vi "FPGA Target 2.vi"() -> ()   [LabVIEW 2025]
uses:
  <vilib>/Platform/TimedLoop/XDataNode/wakeup.ctl
  <vilib>/Platform/TimedLoop/XDataNode/XDNodeRunTimeDep.lvlib
  <vilib>/Platform/TimedLoop/XDataNode/nitl_modes.ctl
  <vilib>/Platform/TimedLoop/XDataNode/timing_clust.ctl
  <vilib>/Platform/TimedLoop/XDataNode/XDataNode.xnode
  SubModules/Engine Simulation Toolkit FPGA IP/IP Source/APU/APU.lvlib
  <vilib>/rvi/DataTransferAndStorage/Container/XNode/niFpgaContainer.xnode
  Templates/FPGA Wizard Templates.lvlib
  <vilib>/rvi/interface/RandomDataEmulation/nirviRandomDataFpgaReadWriteTemplate.vi
  SubModules/Engine Simulation Toolkit FPGA IP/IP Source/Digital Pattern Generation/Digital Pattern Generation.lvlib
  SubModules/Engine Simulation Toolkit FPGA IP/IP Source/Directional Speed/Directional Speed.lvlib
  SubModules/Engine Simulation Toolkit FPGA IP/IP Source/Analog Replay/Analog Replay.lvlib
  SubModules/FPGA Addon Speciality IO/Source/Speciality FPGA IO.lvlib
  SubModules/Engine Simulation Toolkit FPGA IP/IP Source/Knock Sensor/Knock Sensor.lvlib
  SubModules/Engine Simulation Toolkit FPGA IP/IP Source/ECU Event/Timing/ECU Event Timing.lvlib
  SubModules/Engine Simulation Toolkit FPGA IP/IP Source/ECU Event/Timing/Measure Events (Non-40MHz).vi
  SubModules/Engine Simulation Toolkit FPGA IP/IP Source/ECU Event/Timing/Capture Settings.ctl
  SubModules/Engine Simulation Toolkit FPGA IP/IP Source/APU/Shared Settings.ctl
  SubModules/Engine Simulation Toolkit FPGA IP/IP Source/Version Token.ctl
  SubModules/Engine Simulation Toolkit FPGA IP/IP Source/Engine Simulation Toolkit.lvlib
  SubModules/Engine Simulation Toolkit FPGA IP/IP Source/APU/Settings.ctl
  SubModules/Engine Simulation Toolkit FPGA IP/IP Source/APU/Input.ctl
  SubModules/Engine Simulation Toolkit FPGA IP/IP Source/APU/Output.ctl
  SubModules/Engine Simulation Toolkit FPGA IP/IP Source/Digital Pattern Generation/Load Input.ctl
  SubModules/Engine Simulation Toolkit FPGA IP/IP Source/Directional Speed/Load Input.ctl
  SubModules/Engine Simulation Toolkit FPGA IP/IP Source/Analog Replay/Load Input.ctl
  SubModules/FPGA Addon Speciality IO/Source/Types/PWM.Measure.Analog.Settings.ctl
  SubModules/FPGA Addon Speciality IO/Source/Types/PWM.Measure.Analog.Measurement.ctl
  SubModules/Engine Simulation Toolkit FPGA IP/IP Source/Knock Sensor/Cylinder Settings.ctl
  SubModules/Engine Simulation Toolkit FPGA IP/IP Source/Knock Sensor/Cylinder Input.ctl
  SubModules/Engine Simulation Toolkit FPGA IP/IP Source/Knock Sensor/Generate Settings.ctl
  SubModules/Engine Simulation Toolkit FPGA IP/IP Source/Knock Sensor/Generate Input.ctl
  SubModules/Engine Simulation Toolkit FPGA IP/IP Source/Analog Replay/Settings.ctl
  SubModules/Engine Simulation Toolkit FPGA IP/IP Source/Analog Replay/Input.ctl
  SubModules/FPGA Addon Speciality IO/Source/Types/Sine.Generate.Settings.ctl
  SubModules/FPGA Addon Speciality IO/Source/Types/PWM.Generate.Digital.Settings.ctl
  SubModules/Engine Simulation Toolkit FPGA IP/IP Source/Digital Pattern Generation/Settings.ctl
  SubModules/Engine Simulation Toolkit FPGA IP/IP Source/Digital Pattern Generation/Input.ctl
  SubModules/Engine Simulation Toolkit FPGA IP/IP Source/Directional Speed/Settings.ctl
  SubModules/Engine Simulation Toolkit FPGA IP/IP Source/Directional Speed/Input.ctl
  SubModules/FPGA Addon Speciality IO/Source/Types/WSS.Generate.Digital.Settings.ctl
  SubModules/FPGA Addon Speciality IO/Source/Types/PWM.Measure.Digital.Settings.ctl
  SubModules/FPGA Addon Speciality IO/Source/Types/PWM.Measure.Digital.Measurement.ctl
  SubModules/Engine Simulation Toolkit FPGA IP/IP Source/ECU Event/Timing/Measure Settings.ctl
  SubModules/Engine Simulation Toolkit FPGA IP/IP Source/ECU Event/Timing/Measure Output.ctl
  SubModules/Engine Simulation Toolkit FPGA IP/IP Source/ECU Event/Timing/Capture Output.ctl
  SubModules/FPGA Addon Speciality IO/Source/Types/QuadratureEncoder.Measure.Digital.Settings.ctl
  SubModules/FPGA Addon Speciality IO/Source/Types/QuadratureEncoder.Measure.Digital.Measurement.ctl
panel:
  out "Check The Channel 2":bool
  out "Check The Channel 1":bool
  out "Measured CAM Position.Measure":T1
  in  "Measured CAM Position.Settings":T2={"DIRECTION"=0, "RESET VALUE"=0, "A RESET STATE"=TRUE, "B RESET STATE"=TRUE, "Z RESET STATE"=TRUE}
  out "Measured Engine Position.Measure":T1
  in  "Measured Engine Position.Settings":T2={"DIRECTION"=0, "RESET VALUE"=0, "A RESET STATE"=TRUE, "B RESET STATE"=TRUE, "Z RESET STATE"=TRUE}
  out "Connector1 DIO Bank0.Monitor":bool[](array[boolean])
  out "capture.Cyl Inj 3.Event 4":T3
  out "capture.Cyl Inj 3.Event 3":T3
  out "capture.Cyl Inj 3.Event 2":T3
  out "capture.Cyl Inj 3.Event 1":T3
  out "status.Cyl Inj 3":T4
  in  "settings.Cyl Inj 3":T5
  out "capture.Cyl Inj 2.Event 4":T3
  out "capture.Cyl Inj 2.Event 3":T3
  out "capture.Cyl Inj 2.Event 2":T3
  out "capture.Cyl Inj 2.Event 1":T3
  out "status.Cyl Inj 2":T4
  in  "settings.Cyl Inj 2":T5
  out "capture.Cyl Inj 1.Event 4":T3
  out "capture.Cyl Inj 1.Event 3":T3
  out "capture.Cyl Inj 1.Event 2":T3
  out "capture.Cyl Inj 1.Event 1":T3
  out "status.Cyl Inj 1":T4
  in  "settings.Cyl Inj 1":T5
  out "PWM IN 2.Measure":T6
  in  "PWM IN 2.Settings":T7={"ACTIVE EDGE"=TRUE, "TIMEOUT"=40000000}
  out "PWM IN 1.Measure":T6
  in  "PWM IN 1.Settings":T7={"ACTIVE EDGE"=TRUE, "TIMEOUT"=40000000}
  out "Key State":bool
  out "Switch State":bool
  out "Relay State":bool
  out "Connector0 DIO Bank2.Monitor":bool[](array[boolean])
  out "Connector0 DIO Bank1.Monitor":bool[](array[boolean])
  in  "Read Passenger WS.Settings":T8={"ACTIVE EDGE"=TRUE, "ACTIVE TICKS"=0, "INACTIVE TICKS"=0, "DATA"=0, "SENSOR TYPE"=0}
  in  "Rear Driver WS.Settings":T8={"ACTIVE EDGE"=TRUE, "ACTIVE TICKS"=0, "INACTIVE TICKS"=0, "DATA"=0, "SENSOR TYPE"=0}
  in  "Front Passenger WS.Settings":T8={"ACTIVE EDGE"=TRUE, "ACTIVE TICKS"=0, "INACTIVE TICKS"=0, "DATA"=0, "SENSOR TYPE"=0}
  in  "Front Driver WS.Settings":T8={"ACTIVE EDGE"=TRUE, "ACTIVE TICKS"=0, "INACTIVE TICKS"=0, "DATA"=0, "SENSOR TYPE"=0}
  out "Connector0 DIO Bank0.Monitor":bool[](array[boolean])
  in  "input.Crank":T9
  in  "settings.Crank":T10
  in  "input.Crank_Temp":T11
  in  "settings.Crank_Temp":T12
  in  "Switch":bool
  in  "Key":bool
  in  "input.Exhaust CAM 1":T11
  in  "settings.Exhaust CAM 1":T12
  in  "input.Intake CAM 1":T11
  in  "settings.Intake CAM 1":T12
  in  "PWM Out 2.Settings":T13={"ACTIVE EDGE"=TRUE, "ACTIVE TICKS"=0, "INACTIVE TICKS"=0}
  in  "PWM Out 1.Settings":T13={"ACTIVE EDGE"=TRUE, "ACTIVE TICKS"=0, "INACTIVE TICKS"=0}
  out "Connector1 AO Bank0.Monitor":fxp<+/-,32,8>[](array[numeric])
  in  "Simple Knock 2.Settings":T14={"AMP"=0.0, "OFFSET"=0.0, "PERIODS/TICKS"=2.4999957531690598e-05}
  in  "Simple Knock 1.Settings":T14={"AMP"=0.0, "OFFSET"=0.0, "PERIODS/TICKS"=2.4999957531690598e-05}
  in  "input.VR Sensor2":T15
  in  "settings.VR Sensor2":T16
  in  "input.VR Sensor1":T15
  in  "settings.VR Sensor1":T16
  in  "Power Supply Setpoint":fxp<+/-,32,8> format="%#_27g"
  in  "Dyno Setpoint":fxp<+/-,32,8> format="%#_27g"
  in  "input.Knock2":T17
  in  "settings.Knock2":T18
  in  "input.Knock2.Cylinder 6":T19={"probability compare"=65535, "high freq scaler"=0.0, "trigger position"=0}
  in  "settings.Knock2.Cylinder 6":T20
  in  "input.Knock2.Cylinder 5":T19={"probability compare"=65535, "high freq scaler"=0.0, "trigger position"=0}
  in  "settings.Knock2.Cylinder 5":T20
  in  "input.Knock2.Cylinder 4":T19={"probability compare"=65535, "high freq scaler"=0.0, "trigger position"=0}
  in  "settings.Knock2.Cylinder 4":T20
  in  "input.Knock2.Cylinder 3":T19={"probability compare"=65535, "high freq scaler"=0.0, "trigger position"=0}
  in  "settings.Knock2.Cylinder 3":T20
  in  "input.Knock2.Cylinder 2":T19={"probability compare"=65535, "high freq scaler"=0.0, "trigger position"=0}
  in  "settings.Knock2.Cylinder 2":T20
  in  "input.Knock2.Cylinder 1":T19={"probability compare"=65535, "high freq scaler"=0.0, "trigger position"=0}
  in  "settings.Knock2.Cylinder 1":T20
  in  "input.Knock1":T17
  in  "settings.Knock1":T18
  in  "input.Knock1.Cylinder 6":T19={"probability compare"=65535, "high freq scaler"=0.0, "trigger position"=0}
  in  "settings.Knock1.Cylinder 6":T20
  in  "input.Knock1.Cylinder 5":T19={"probability compare"=65535, "high freq scaler"=0.0, "trigger position"=0}
  in  "settings.Knock1.Cylinder 5":T20
  in  "input.Knock1.Cylinder 4":T19={"probability compare"=65535, "high freq scaler"=0.0, "trigger position"=0}
  in  "settings.Knock1.Cylinder 4":T20
  in  "input.Knock1.Cylinder 3":T19={"probability compare"=65535, "high freq scaler"=0.0, "trigger position"=0}
  in  "settings.Knock1.Cylinder 3":T20
  in  "input.Knock1.Cylinder 2":T19={"probability compare"=65535, "high freq scaler"=0.0, "trigger position"=0}
  in  "settings.Knock1.Cylinder 2":T20
  in  "input.Knock1.Cylinder 1":T19={"probability compare"=65535, "high freq scaler"=0.0, "trigger position"=0}
  in  "settings.Knock1.Cylinder 1":T20
  out "Temp2":fxp<+/-,32,8> format="%#_27g"
  out "Temp1":fxp<+/-,32,8> format="%#_27g"
  out "Pressure4":fxp<+/-,32,8> format="%#_27g"
  out "Pressure3":fxp<+/-,32,8> format="%#_27g"
  out "Injector4.Measure":T21
  in  "Injector4.Settings":T22={"ACTIVE EDGE"=TRUE, "TIMEOUT"=40000000, "THRESHOLD"=50.0}
  out "Injector3.Measure":T21
  in  "Injector3.Settings":T22={"ACTIVE EDGE"=TRUE, "TIMEOUT"=40000000, "THRESHOLD"=50.0}
  out "Pressure2":fxp<+/-,32,8> format="%#_27g"
  out "Pressure1":fxp<+/-,32,8> format="%#_27g"
  out "Connector1 AI Bank0.Monitor":fxp<+/-,27,5>[](array[numeric])
  in  "load input.VR Sensor2":T23={"Data"=[0, 0, 0, 0, 0, 0, 0, 0, 0, 0, 0, 0, 0, 0, 0, 0], "LoadOffset"=0, "Done"=FALSE}
  in  "load input.VR Sensor1":T23={"Data"=[0, 0, 0, 0, 0, 0, 0, 0, 0, 0, 0, 0, 0, 0, 0, 0], "LoadOffset"=0, "Done"=FALSE}
  in  "load input.Crank":T24
  in  "load input.Crank_Temp":T25
  in  "load input.Exhaust CAM 1":T25
  in  "load input.Intake CAM 1":T25
  out "Actual Analog Input Loop Period (usec)":u32
  out "Actual Analog Output Loop Period (usec)":u32
  out "Actual Digital Loop Period (usec)":u32
  out "Actual DMA Loop Period (usec)":u32
  in  "Analog Input Loop Timer (uSec)":u32=10
  out "output.apu 1":T26 caption="output"
  in  "input.apu 1":T27={"desired speed"=0.0, "reset"=TRUE} caption="input"
  in  "settings.apu 1":T28 caption="settings"
  in  "est.version":T29
  in  "shared settings.apu 1":T30 {"start" format="%#.15g"}
  in  "go.apu 1":bool
  in  "Digital Loop Timer (uSec)":u32=10
  in  "Analog Output Loop Timer (uSec)":u32=10
  in  "DMA.Enable":bool
  in  "DMA.MinimumSamples":u32=100000 caption="DMA Loop Timer (uSec)"
  out "DMA.Timeout":bool
  in  "DMA.Timeout.Reset":bool
  in  "DMA Loop Timer (uSec)":u32=10
types:
  T1 = typedef "Speciality FPGA IO.lvlib/QuadratureEncoder.Measure.Digital.Measurement.ctl" = cluster{"POSITION":i32}
  T2 = typedef "Speciality FPGA IO.lvlib/QuadratureEncoder.Measure.Digital.Settings.ctl" = cluster{"DIRECTION":u8, "RESET VALUE":i32, "A RESET STATE":bool, "B RESET STATE":bool, "Z RESET STATE":bool}
  T3 = typedef "Engine Simulation Toolkit.lvlib/ECU Event Timing.lvlib/Capture Output.ctl" = cluster{"Start":u16, "End":u16, "Duration (tics)":fxp<+,18,18>, "Event present":bool}
  T4 = typedef "Engine Simulation Toolkit.lvlib/ECU Event Timing.lvlib/Measure Output.ctl" = cluster{"stuck active":bool, "window all active":bool, "window orphan start":bool, "window orphan end":bool}
  T5 = typedef "Engine Simulation Toolkit.lvlib/ECU Event Timing.lvlib/Measure Settings.ctl" = cluster{"max":u16, "min":u16, "active high":bool, "wrap":bool}
  T6 = typedef "Speciality FPGA IO.lvlib/PWM.Measure.Digital.Measurement.ctl" = cluster{"ACTIVE TICKS":u32, "INACTIVE TICKS":u32, "ACQ TICKS":u32}
  T7 = typedef "Speciality FPGA IO.lvlib/PWM.Measure.Digital.Settings.ctl" = cluster{"ACTIVE EDGE":bool, "TIMEOUT":u32}
  T8 = typedef "Speciality FPGA IO.lvlib/WSS.Generate.Digital.Settings.ctl" = cluster{"ACTIVE EDGE":bool, "ACTIVE TICKS":u32, "INACTIVE TICKS":u32, "DATA":u8, "SENSOR TYPE":u8}
  T9 = typedef "Engine Simulation Toolkit.lvlib/Directional Speed.lvlib/Input.ctl" = cluster{"td (tics)":u16, "tf (tics)":u16, "tr (tics)":u16}
  T10 = typedef "Engine Simulation Toolkit.lvlib/Directional Speed.lvlib/Settings.ctl" = cluster{"Upper Value":u16, "Lower Value":u16, "Upper Index":fxp<+,10,10>, "Lower Index":fxp<+,10,10>, "Enabled":bool}
  T11 = typedef "Engine Simulation Toolkit.lvlib/Digital Pattern Generation.lvlib/Input.ctl" = cluster{"Offset":i16}
  T12 = typedef "Engine Simulation Toolkit.lvlib/Digital Pattern Generation.lvlib/Settings.ctl" = cluster{"edge 1":u16, "edge 2":u16, "cycle angle":bool, "enabled":bool, "first falling":bool, "fault":bool, "fault wrap":bool, "fault value":bool, "fault count":fxp<+,4,4>, "use fault count":bool}
  T13 = typedef "Speciality FPGA IO.lvlib/PWM.Generate.Digital.Settings.ctl" = cluster{"ACTIVE EDGE":bool, "ACTIVE TICKS":u32, "INACTIVE TICKS":u32}
  T14 = typedef "Speciality FPGA IO.lvlib/Sine.Generate.Settings.ctl" = cluster{"AMP":fxp<+/-,32,8>, "OFFSET":fxp<+/-,32,8>, "PERIODS/TICKS":fxp<+,32,0>}
  T15 = typedef "Engine Simulation Toolkit.lvlib/Analog Replay.lvlib/Input.ctl" = cluster{"Offset":i16, "VScaleSlope":fxp<+,18,6>, "VScaleIntercept":fxp<+/-,18,3>}
  T16 = typedef "Engine Simulation Toolkit.lvlib/Analog Replay.lvlib/Settings.ctl" = cluster{"ReverseNegate":bool, "CycleAngle":bool, "SpeedThreshold":fxp<+/-,23,2>, "AOBelowThreshold":i16}
  T17 = typedef "Engine Simulation Toolkit.lvlib/Knock Sensor.lvlib/Generate Input.ctl" = cluster{"low freq scaler":fxp<+,10,0>}
  T18 = typedef "Engine Simulation Toolkit.lvlib/Knock Sensor.lvlib/Generate Settings.ctl" = cluster{"low freq (periods/tick)":fxp<+,32,0>, "high freq (periods/tick)":fxp<+,32,0>, "duration (1.25MHz tics)":fxp<+,18,18>, "low freq speed slope":fxp<+,16,-3>, "low freq speed intercept":fxp<+,10,-10>, "low freq by speed":bool}
  T19 = typedef "Engine Simulation Toolkit.lvlib/Knock Sensor.lvlib/Cylinder Input.ctl" = cluster{"probability compare":u16, "high freq scaler":fxp<+,10,0>, "trigger position":u16}
  T20 = typedef "Engine Simulation Toolkit.lvlib/Knock Sensor.lvlib/Cylinder Settings.ctl" = cluster{"seed":u16, "reset":bool}
  T21 = typedef "Speciality FPGA IO.lvlib/PWM.Measure.Analog.Measurement.ctl" = cluster{"ACTIVE TICKS":u32, "INACTIVE TICKS":u32, "ACQ TICKS":u32, "ACTIVE VOLTAGE":fxp<+/-,32,8>, "INACTIVE VOLTAGE":fxp<+/-,32,8>}
  T22 = typedef "Speciality FPGA IO.lvlib/PWM.Measure.Analog.Settings.ctl" = cluster{"ACTIVE EDGE":bool, "TIMEOUT":u32, "THRESHOLD":fxp<+/-,32,8>}
  T23 = typedef "Engine Simulation Toolkit.lvlib/Analog Replay.lvlib/Load Input.ctl" = cluster{"Data":i16[], "LoadOffset":u16, "Done":bool}
  T24 = typedef "Engine Simulation Toolkit.lvlib/Directional Speed.lvlib/Load Input.ctl" = cluster{"address":fxp<+,10,10>, "done":bool, "angle":u16}
  T25 = typedef "Engine Simulation Toolkit.lvlib/Digital Pattern Generation.lvlib/Load Input.ctl" = cluster{"address":fxp<+,11,11>, "done":bool, "angle":u16}
  T26 = typedef "Engine Simulation Toolkit.lvlib/APU.lvlib/Output.ctl" = cluster{"crank":u16, "cycle":u16, "actual speed":fxp<+/-,23,2>}
  T27 = typedef "Engine Simulation Toolkit.lvlib/APU.lvlib/Input.ctl" = cluster{"desired speed":fxp<+/-,23,2>, "reset":bool}
  T28 = typedef "Engine Simulation Toolkit.lvlib/APU.lvlib/Settings.ctl" = cluster{"acceleration":fxp<+,18,-20>, "enable accel":bool}
  T29 = typedef "Engine Simulation Toolkit.lvlib/Version Token.ctl" = cluster{"1.4.0":bool}
  T30 = typedef "Engine Simulation Toolkit.lvlib/APU.lvlib/Shared Settings.ctl" = cluster{"start":fxp<+,17,17>, "stuck limit":fxp<+,18,18>}
  T31 = typedef "XDNodeRunTimeDep.lvlib/timing_clust.ctl" = cluster{"Expected End [f-1]":u64, "Actual End [f-1]":u64, "Finished Late? [f-1]":bool, "Expected End [i-1]":u64, "Actual End [i-1]":u64, "Finished Late? [i-1]":bool, "Expected Start [i]":u64, "Actual Start [i]":u64, "Expected Start [f]":u64, "Actual Start [f]":u64, "Source Name":string, "Structure Name":string, "Period":i64, "Deadline":i64, "Offset":i64, "Start":i64, "Priority":i32, "Timeout":i32, "Mode":T32, "Wakeup Reason":T33, "Error":errorcluster, "Source Type":string, "Secondary Source Type":string, "Global End Time":u64, "Global Start Time":u64, "Frame Duration":u64, "Iteration Duration":u64, "Assigned CPU":i32, "I/O Scan Engine Mode":u32}
  T32 = typedef "XDNodeRunTimeDep.lvlib/nitl_modes.ctl" = enum32{"No Change", "Process missed periods, maintain original phase", "Discard missed periods, maintain original phase", "Process missed periods, ignore original phase", "Discard missed periods, ignore original phase"}
  T33 = typedef "XDNodeRunTimeDep.lvlib/wakeup.ctl" = enum32{"Normal", "Aborted", "Asynchronous wakeup", "Timing source error", "Timed loop error", "Timeout"}
  T34 = cluster{"DI 0":refnum<k21>, "DI 1":refnum<k21>, "DI 2":refnum<k21>, "DI 3":refnum<k21>, "DI 4":refnum<k21>, "DI 5":refnum<k21>, "DI 6":refnum<k21>, "DI 7":refnum<k21>}
  T35 = typedef "Engine Simulation Toolkit.lvlib/ECU Event Timing.lvlib/Capture Settings.ctl" = u8
  T36 = cluster{"DO 0":refnum<k21>, "DO 1":refnum<k21>, "DO 2":refnum<k21>, "DO 3":refnum<k21>, "DO 4":refnum<k21>, "DO 5":refnum<k21>, "DO 6":refnum<k21>, "DO 7":refnum<k21>}
  T37 = cluster{"AO 0":refnum<k21>, "AO 1":refnum<k21>, "AO 2":refnum<k21>, "AO 3":refnum<k21>, "AO 4":refnum<k21>, "AO 5":refnum<k21>, "AO 6":refnum<k21>, "AO 7":refnum<k21>}
  T38 = cluster{"AI 0":refnum<k21>, "AI 1":refnum<k21>, "AI 2":refnum<k21>, "AI 3":refnum<k21>, "AI 4":refnum<k21>, "AI 5":refnum<k21>, "AI 6":refnum<k21>, "AI 7":refnum<k21>}
  T39 = typedef "Engine Simulation Toolkit.lvlib/Digital Pattern Generation.lvlib/Load Data.ctl" = cluster{"max address":fxp<+,11,11>, "memory":refnum<k21>}
  T40 = typedef "Engine Simulation Toolkit.lvlib/Directional Speed.lvlib/Load Data.ctl" = cluster{"max address":fxp<+,10,10>, "Memory":refnum<k21>}
  T41 = typedef "Engine Simulation Toolkit.lvlib/APU.lvlib/Register Bus.ctl" = cluster{"Speed":refnum<k21>, "Crank Angle":refnum<k21>, "Cycle Angle":refnum<k21>, "Crank Count":refnum<k21>, "Cycle Count":refnum<k21>, "1.25 MHz Counter":refnum<k21>, "Crank Rollover":refnum<k21>, "Cycle Rollover":refnum<k21>, "shared settings":T30}
  T42 = typedef "Engine Simulation Toolkit.lvlib/Knock Sensor.lvlib/Triggered Cylinder Data.ctl" = cluster{"trigger knock":bool, "high freq scaler":fxp<+,10,0>}
  T43 = typedef "Engine Simulation Toolkit.lvlib/ECU Event Timing.lvlib/Measured Data.ctl" = cluster{"start":u16, "end":u16, "duration (tics)":fxp<+,18,18>, "window end":bool, "window begin":bool, "pulse end":bool, "pulse #":u8}
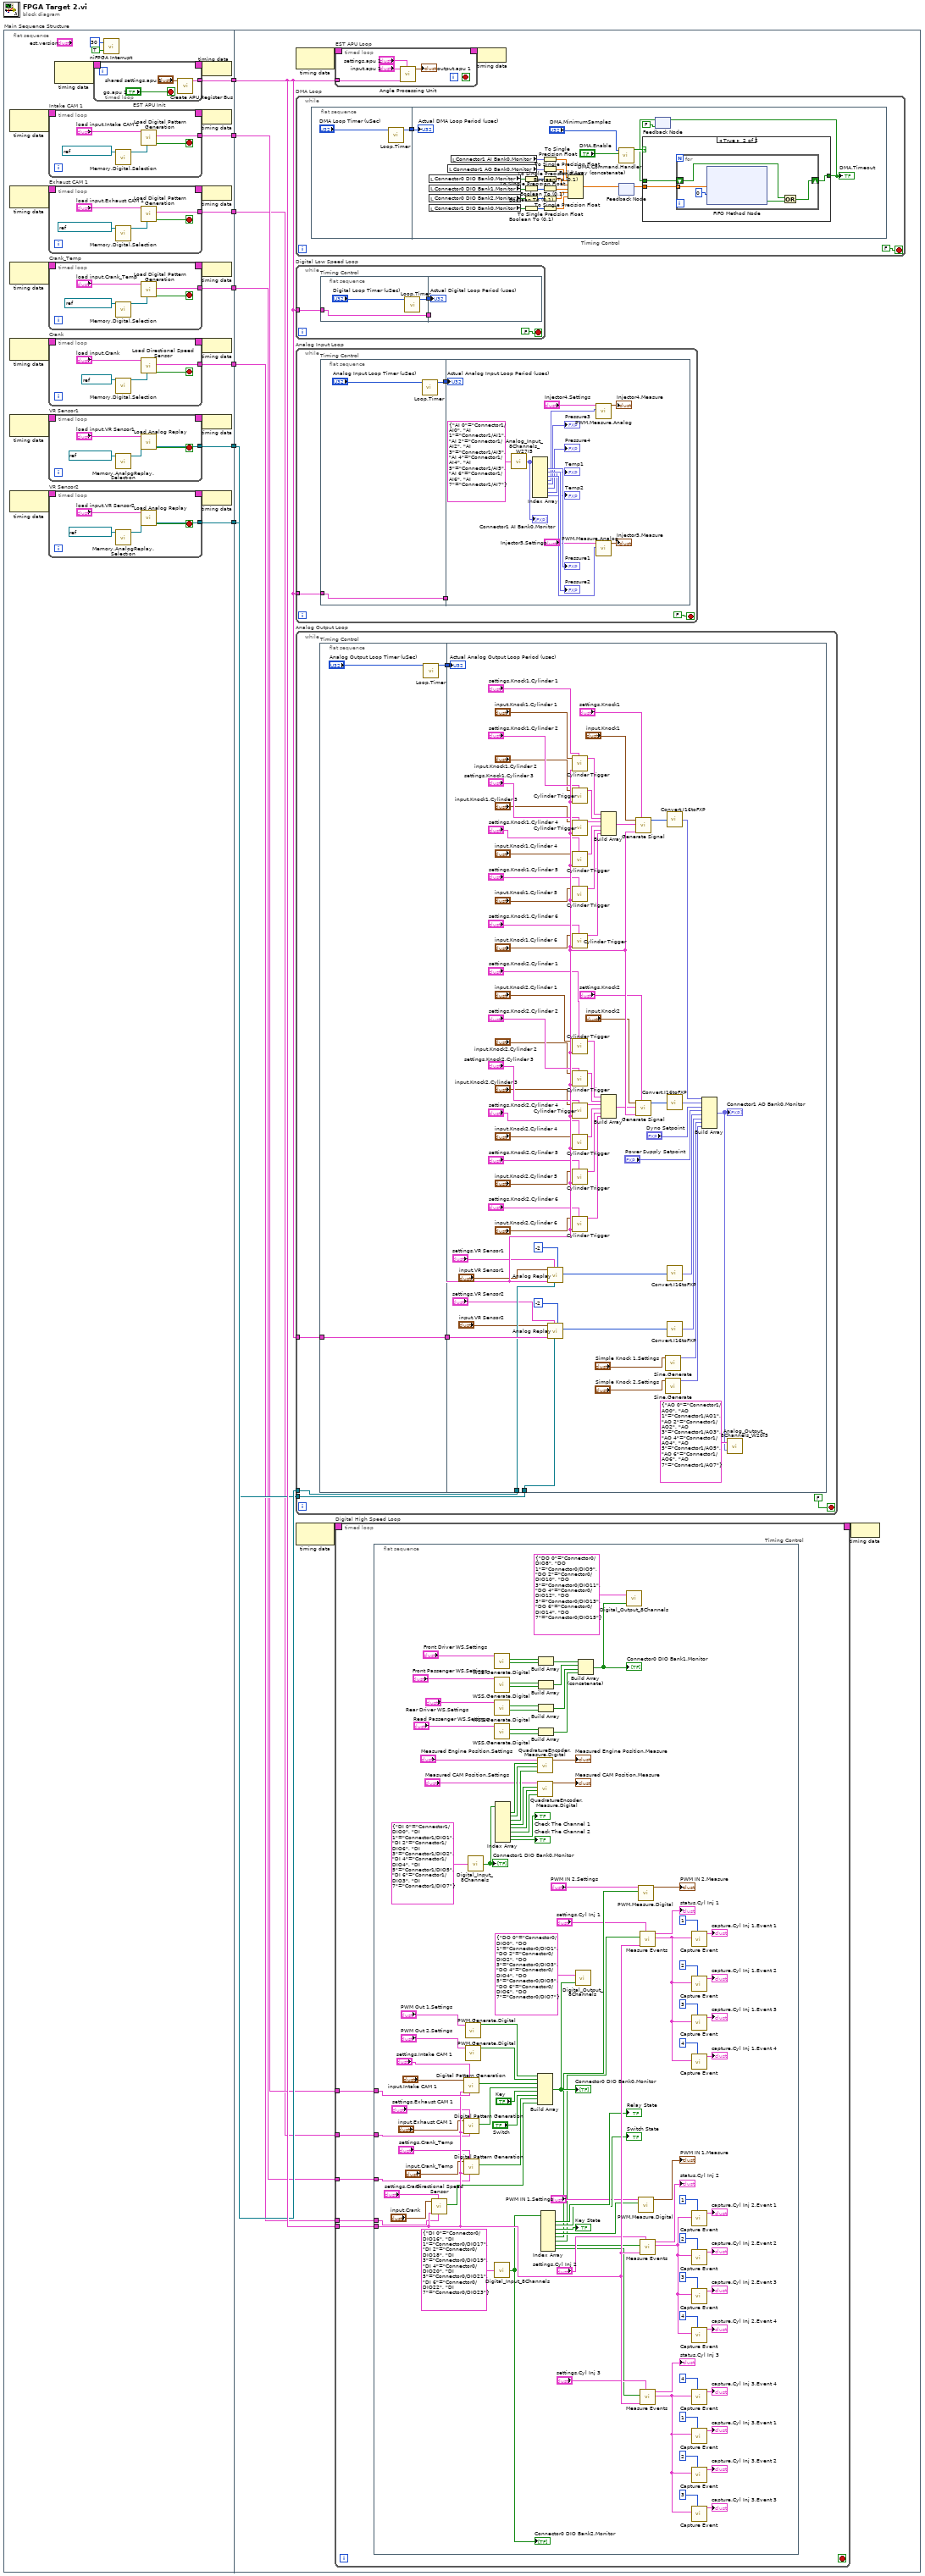
[diagram p0: block diagram]
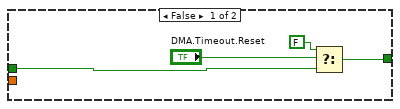
[diagram p2: hidden frame]
diagram:
  n1 = flat-sequence "Main Sequence Structure" {
    tunnel: [w26] -> w7
    tunnel: [w13] -> w6
    tunnel: [w12] -> w5
    tunnel: [w11] -> w4
    tunnel: [w10] -> w3
    tunnel: [w9] -> w2
    tunnel: [w8] -> w1
    tunnel: w7 -> [w96]
    tunnel: w6 -> [w95]
    tunnel: w5 -> [w94]
    tunnel: w4 -> [w93]
    tunnel: w3 -> [w92]
    tunnel: w2 -> [w91]
    tunnel: w1 -> [w90]
    frame #0 {
      n2 = node-c288() -> (w25:T31)  [unwired: 1 in]
      n3 = node-c288() -> (w23:T31)  [unwired: 1 in]
      n4 = node-c288() -> (w21:T31)  [unwired: 1 in]
      n5 = node-c288() -> (w19:T31)  [unwired: 1 in]
      n6 = node-c288() -> (w17:T31)  [unwired: 1 in]
      n7 = node-c288() -> (w15:T31)  [unwired: 1 in]
      n8 = timed-loop "Intake CAM 1" {
        timing: w25 -> [_]
        timing-out: [_] -> w24
        tunnel: [w74] -> w11
        stop <- w77 stop-if-true
        n9 = call "Memory.Digital.Selection.vi"("memory"=refnum<k21> "Intake CAM 1") -> ("memory"=w75:refnum<k21>)  [unwired: 10 in]
        n10 = call "Load Digital Pattern Generation.vi"("memory"=w75, "load input.<user name>"="load input.Intake CAM 1") -> ("done"=w77:bool, "load data"=w74:T39)  [unwired: 8 in]
      }
      n11 = timed-loop "Exhaust CAM 1" {
        timing: w23 -> [_]
        timing-out: [_] -> w22
        tunnel: [w65] -> w10
        stop <- w68 stop-if-true
        n12 = call "Memory.Digital.Selection.vi"("memory"=refnum<k21> "Exhaust CAM 1") -> ("memory"=w66:refnum<k21>)  [unwired: 10 in]
        n13 = call "Load Digital Pattern Generation.vi"("memory"=w66, "load input.<user name>"="load input.Exhaust CAM 1") -> ("done"=w68:bool, "load data"=w65:T39)  [unwired: 8 in]
      }
      n14 = timed-loop "Crank_Temp" {
        timing: w21 -> [_]
        timing-out: [_] -> w20
        tunnel: [w56] -> w9
        stop <- w59 stop-if-true
        n15 = call "Memory.Digital.Selection.vi"("memory"=refnum<k21> "Crank_Temp") -> ("memory"=w57:refnum<k21>)  [unwired: 10 in]
        n16 = call "Load Digital Pattern Generation.vi"("memory"=w57, "load input.<user name>"="load input.Crank_Temp") -> ("done"=w59:bool, "load data"=w56:T39)  [unwired: 8 in]
      }
      n17 = timed-loop "Crank" {
        timing: w19 -> [_]
        timing-out: [_] -> w18
        tunnel: [w47] -> w8
        stop <- w50 stop-if-true
        n18 = call "Memory.Digital.Selection.vi"("memory"=refnum<k21> "Crank") -> ("memory"=w48:refnum<k21>)  [unwired: 10 in]
        n19 = call "Load Directional Speed Sensor.vi"("Memory In"=w48, "load input.<user name>"="load input.Crank") -> ("done"=w50:bool, "load data"=w47:T40)  [unwired: 8 in]
      }
      n20 = timed-loop "VR Sensor1" {
        timing: w17 -> [_]
        timing-out: [_] -> w16
        tunnel: [w39] -> w13
        stop <- w41 stop-if-true
        n21 = call "Memory.AnalogReplay.Selection.vi"("memory"=refnum<k21> "VR Sensor1") -> ("memory"=w39:refnum<k21>)  [unwired: 10 in]
        n22 = call "Load Analog Replay.vi"("memory"=w39, "load input.<user name>"="load input.VR Sensor1") -> ("done"=w41:bool)  [unwired: 9 in]
      }
      n23 = timed-loop "VR Sensor2" {
        timing: w15 -> [_]
        timing-out: [_] -> w14
        tunnel: [w31] -> w12
        stop <- w33 stop-if-true
        n24 = call "Memory.AnalogReplay.Selection.vi"("memory"=refnum<k21> "VR Sensor2") -> ("memory"=w31:refnum<k21>)  [unwired: 10 in]
        n25 = call "Load Analog Replay.vi"("memory"=w31, "load input.<user name>"="load input.VR Sensor2") -> ("done"=w33:bool)  [unwired: 9 in]
      }
      n26 = node-c288() -> (w28:T31)  [unwired: 1 in]
      n27 = timed-loop "EST APU Init" {
        timing: w28 -> [_]
        timing-out: [_] -> w27
        tunnel: [w83] -> w26
        stop <- "go.apu 1" stop-if-true
        n28 = call "Create APU Register Bus.vi"("shared settings.<user name>"="shared settings.apu 1") -> ("register bus"=w83:T41)  [unwired: 10 in]
      }
      n29 = call <vilib>:"niFPGA Interrupt.vi"("Wait Until Cleared (F)"=TRUE, "IRQ Number (0)"=u8 30) -> ()  [unwired: 1 in]
      n30 = node-c288(w27) -> ()
      n31 = node-c288(w24) -> ()
      n32 = node-c288(w22) -> ()
      n33 = node-c288(w20) -> ()
      n34 = node-c288(w18) -> ()
      n35 = node-c288(w16) -> ()
      n36 = node-c288(w14) -> ()
    }
    frame #1 {
      # "FPGA Addon Code"
      n37 = node-c288 ("Input Node")() -> (w98:T31)  [unwired: 1 in]
      n38 = while "DMA Loop" {
        stop <- FALSE stop-if-true
        n39 = flat-sequence "Timing Control" {
          tunnel: [w224] -> w222
          tunnel: w222 -> [w242]
          frame #0 {
            n40 = call "Loop.Timer.vi"("Loop Timer (uSec)"="DMA Loop Timer (uSec)") -> ("Actual Loop Period (usec)"=w224:u32)  [unwired: 10 in]
          }
          frame #1 {
            n41 = local read "Connector0 DIO Bank0.Monitor"() -> (w239:bool[])
            n42 = local read "Connector0 DIO Bank1.Monitor"() -> (w237:bool[])
            n43 = local read "Connector0 DIO Bank2.Monitor"() -> (w235:bool[])
            n44 = local read "Connector1 DIO Bank0.Monitor"() -> (w233:bool[])
            n45 = local read "Connector1 AO Bank0.Monitor"() -> (w240:fxp<+/-,32,8>[])
            n46 = local read "Connector1 AI Bank0.Monitor"() -> (w241:fxp<+/-,27,5>[])
            n47 = Boolean To (0,1)(Boolean=w239) -> (0, 1=w238:i16[])
            n48 = Boolean To (0,1)(Boolean=w237) -> (0, 1=w236:i16[])
            n49 = Boolean To (0,1)(Boolean=w235) -> (0, 1=w234:i16[])
            n50 = Boolean To (0,1)(Boolean=w233) -> (0, 1=w232:i16[])
            n51 = To Single Precision Float(number=w241) -> (single precision float=w231:sgl[])
            n52 = To Single Precision Float(number=w240) -> (single precision float=w230:sgl[])
            n53 = To Single Precision Float(number=w238) -> (single precision float=w229:sgl[])
            n54 = To Single Precision Float(number=w236) -> (single precision float=w228:sgl[])
            n55 = To Single Precision Float(number=w234) -> (single precision float=w227:sgl[])
            n56 = To Single Precision Float(number=w232) -> (single precision float=w226:sgl[])
            n57 = Build Array (concatenate) "Build Array"(w231, w230, w229, w228, w227, w226) -> (w248:sgl[])
            n58 = call "DMA.Command.Handler.vi"("DMA.Enable"="DMA.Enable", "DMA.MinimumSamples"="DMA.MinimumSamples") -> ("Transfer"=w244:bool)  [unwired: 9 in]
            n59 = feedback #1() -> (w247:sgl[])  [unwired: 1 in]
            n60 = feedback-in #1(w248) -> ()
            n61 = feedback #2(FALSE ("t")) -> (w243:bool)
            n62 = case shown="True" w244 {
              tunnel: w247 -> [_ w257]
              tunnel: w243 -> [w252 w256]
              tunnel: [w251 w255] -> w246
              frame False {
                n63 = Select(t=FALSE, s="DMA.Timeout.Reset", f=w252) -> (s? t:f=w251:bool)
              }
              frame True {
                n64 = for {
                  shift-right: [w260] -> w255
                  shift-left: w256 -> [w259]
                  tunnel: w257 -> [w258] mode=indexing
                  n65 = xnode ("FIFO Method Node")("Element"=w258, "Timeout"=0) -> ("Timed Out?"=w261:bool)  [unwired: 1 in, 1 out]
                  n66 = Or(x=w259, y=w261) -> (x .or. y?=w260:bool)
                }
              }
            }
            "DMA.Timeout" <- w246
            n67 = feedback-in #2(w246) -> ()
            "Actual DMA Loop Period (usec)" <- w242
          }
        }
      }
      n68 = while "Digital Low Speed Loop" {
        tunnel: w96 -> [w364]
        stop <- FALSE stop-if-true
        n69 = flat-sequence "Timing Control" {
          tunnel: w364 -> [w368]
          tunnel: [w368] -> w363
          tunnel: [w366] -> w362
          tunnel: w363 -> [_]
          tunnel: w362 -> [w369]
          frame #0 {
            n70 = call "Loop.Timer.vi"("Loop Timer (uSec)"="Digital Loop Timer (uSec)") -> ("Actual Loop Period (usec)"=w366:u32)  [unwired: 10 in]
          }
          frame #1 {
            "Actual Digital Loop Period (usec)" <- w369
          }
        }
      }
      n71 = while "Analog Input Loop" {
        tunnel: w96 -> [w342]
        stop <- FALSE stop-if-true
        n72 = flat-sequence "Timing Control" {
          tunnel: w342 -> [w346]
          tunnel: [w346] -> w341
          tunnel: [w344] -> w340
          tunnel: w341 -> [_]
          tunnel: w340 -> [w361]
          frame #0 {
            n73 = call "Loop.Timer.vi"("Loop Timer (uSec)"="Analog Input Loop Timer (uSec)") -> ("Actual Loop Period (usec)"=w344:u32)  [unwired: 10 in]
          }
          frame #1 {
            n74 = call "Analog_Input_8Channels_W27I5.vi"("IO"=T38 {"AI 0"="Connector1/AI0", "AI 1"="Connector1/AI1", "AI 2"="Connector1/AI2", "AI 3"="Connector1/AI3", "AI 4"="Connector1/AI4", "AI 5"="Connector1/AI5", "AI 6"="Connector1/AI6", "AI 7"="Connector1/AI7"}) -> ("Values"=w359:fxp<+/-,27,5>[])
            "Connector1 AI Bank0.Monitor" <- w359
            n75 = Index Array(array=w359) -> (element #1=→"Pressure1":fxp<+/-,27,5>, element #2=→"Pressure2":fxp<+/-,27,5>, element #3=w355:fxp<+/-,27,5>, element #4=w352:fxp<+/-,27,5>, element #5=→"Pressure3":fxp<+/-,27,5>, element #6=→"Pressure4":fxp<+/-,27,5>, element #7=→"Temp1":fxp<+/-,27,5>, element #8=→"Temp2":fxp<+/-,27,5>)  [unwired: 8 in]
            n76 = call "PWM.Measure.Analog.vi"("PWM"=w352, "Settings"="Injector4.Settings") -> ("Measurement"=→"Injector4.Measure":T21)  [unwired: 8 in, 1 out]
            n77 = call "PWM.Measure.Analog.vi"("PWM"=w355, "Settings"="Injector3.Settings") -> ("Measurement"=→"Injector3.Measure":T21)  [unwired: 8 in, 1 out]
            "Actual Analog Input Loop Period (usec)" <- w361
          }
        }
      }
      n78 = while "Analog Output Loop" {
        tunnel: w96 -> [w267]
        tunnel: w95 -> [w264]
        tunnel: w94 -> [w263]
        stop <- FALSE stop-if-true
        n79 = flat-sequence "Timing Control" {
          tunnel: w267 -> [w271]
          tunnel: [w271] -> w266
          tunnel: [w269] -> w265
          tunnel: w266 -> [w336]
          tunnel: w265 -> [w339]
          tunnel: w264 -> [w290]
          tunnel: w263 -> [w285]
          frame #0 {
            n80 = call "Loop.Timer.vi"("Loop Timer (uSec)"="Analog Output Loop Timer (uSec)") -> ("Actual Loop Period (usec)"=w269:u32)  [unwired: 10 in]
          }
          frame #1 {
            n81 = call "Analog Replay.vi"("shift"=i8 -2, "memory"=w290, "settings.<user name>"="settings.VR Sensor1", "register bus"=w336, "input.<user name>"="input.VR Sensor1") -> ("analog value"=w289:i16)  [unwired: 6 in]
            n82 = call "Analog Replay.vi"("shift"=i8 -2, "memory"=w285, "settings.<user name>"="settings.VR Sensor2", "register bus"=w336, "input.<user name>"="input.VR Sensor2") -> ("analog value"=w284:i16)  [unwired: 6 in]
            n83 = call "Cylinder Trigger.vi"("settings.<user name>"="settings.Knock1.Cylinder 1", "register bus"=w336, "input.<user name>"="input.Knock1.Cylinder 1") -> ("triggered knock data"=w335:T42)  [unwired: 8 in]
            n84 = call "Cylinder Trigger.vi"("settings.<user name>"="settings.Knock1.Cylinder 2", "register bus"=w336, "input.<user name>"="input.Knock1.Cylinder 2") -> ("triggered knock data"=w332:T42)  [unwired: 8 in]
            n85 = call "Cylinder Trigger.vi"("settings.<user name>"="settings.Knock1.Cylinder 3", "register bus"=w336, "input.<user name>"="input.Knock1.Cylinder 3") -> ("triggered knock data"=w329:T42)  [unwired: 8 in]
            n86 = call "Cylinder Trigger.vi"("settings.<user name>"="settings.Knock1.Cylinder 4", "register bus"=w336, "input.<user name>"="input.Knock1.Cylinder 4") -> ("triggered knock data"=w326:T42)  [unwired: 8 in]
            n87 = call "Cylinder Trigger.vi"("settings.<user name>"="settings.Knock1.Cylinder 5", "register bus"=w336, "input.<user name>"="input.Knock1.Cylinder 5") -> ("triggered knock data"=w323:T42)  [unwired: 8 in]
            n88 = call "Cylinder Trigger.vi"("settings.<user name>"="settings.Knock1.Cylinder 6", "register bus"=w336, "input.<user name>"="input.Knock1.Cylinder 6") -> ("triggered knock data"=w320:T42)  [unwired: 8 in]
            n89 = call "Cylinder Trigger.vi"("settings.<user name>"="settings.Knock2.Cylinder 1", "register bus"=w336, "input.<user name>"="input.Knock2.Cylinder 1") -> ("triggered knock data"=w313:T42)  [unwired: 8 in]
            n90 = call "Cylinder Trigger.vi"("settings.<user name>"="settings.Knock2.Cylinder 2", "register bus"=w336, "input.<user name>"="input.Knock2.Cylinder 2") -> ("triggered knock data"=w310:T42)  [unwired: 8 in]
            n91 = call "Cylinder Trigger.vi"("settings.<user name>"="settings.Knock2.Cylinder 3", "register bus"=w336, "input.<user name>"="input.Knock2.Cylinder 3") -> ("triggered knock data"=w307:T42)  [unwired: 8 in]
            n92 = call "Cylinder Trigger.vi"("settings.<user name>"="settings.Knock2.Cylinder 4", "register bus"=w336, "input.<user name>"="input.Knock2.Cylinder 4") -> ("triggered knock data"=w304:T42)  [unwired: 8 in]
            n93 = call "Cylinder Trigger.vi"("settings.<user name>"="settings.Knock2.Cylinder 5", "register bus"=w336, "input.<user name>"="input.Knock2.Cylinder 5") -> ("triggered knock data"=w301:T42)  [unwired: 8 in]
            n94 = call "Cylinder Trigger.vi"("settings.<user name>"="settings.Knock2.Cylinder 6", "register bus"=w336, "input.<user name>"="input.Knock2.Cylinder 6") -> ("triggered knock data"=w298:T42)  [unwired: 8 in]
            n95 = Build Array(w335, w332, w329, w326, w323, w320) -> (w317:T42[])
            n96 = Build Array(w313, w310, w307, w304, w301, w298) -> (w295:T42[])
            n97 = call "Generate Signal.vi"("settings.<user name>"="settings.Knock1", "register bus"=w336, "triggered knock data"=w317, "input.<user name>"="input.Knock1") -> ("knock signal"=w316:i16)  [unwired: 7 in]
            n98 = call "Generate Signal.vi"("settings.<user name>"="settings.Knock2", "register bus"=w336, "triggered knock data"=w295, "input.<user name>"="input.Knock2") -> ("knock signal"=w294:i16)  [unwired: 7 in]
            n99 = call "Sine.Generate.vi"("Settings"="Simple Knock 1.Settings") -> ("Output"=w275:fxp<+/-,32,8>)  [unwired: 10 in]
            n100 = call "Sine.Generate.vi"("Settings"="Simple Knock 2.Settings") -> ("Output"=w274:fxp<+/-,32,8>)  [unwired: 10 in]
            n101 = call "Convert.I16toFXP.vi"("16bit integer"=w316) -> ("x*y"=w281:fxp<+/-,20,5>)  [unwired: 4 in]
            n102 = call "Convert.I16toFXP.vi"("16bit integer"=w294) -> ("x*y"=w280:fxp<+/-,20,5>)  [unwired: 4 in]
            n103 = call "Convert.I16toFXP.vi"("16bit integer"=w289) -> ("x*y"=w277:fxp<+/-,20,5>)  [unwired: 4 in]
            n104 = call "Convert.I16toFXP.vi"("16bit integer"=w284) -> ("x*y"=w276:fxp<+/-,20,5>)  [unwired: 4 in]
            n105 = Build Array(w281, w280, "Dyno Setpoint", "Power Supply Setpoint", w277, w276, w275, w274) -> (w272:fxp<+/-,32,8>[])
            "Connector1 AO Bank0.Monitor" <- w272
            n106 = call "Analog_Output_8Channels_W20I5.vi"("Values"=w272, "IO"=T37 {"AO 0"="Connector1/AO0", "AO 1"="Connector1/AO1", "AO 2"="Connector1/AO2", "AO 3"="Connector1/AO3", "AO 4"="Connector1/AO4", "AO 5"="Connector1/AO5", "AO 6"="Connector1/AO6", "AO 7"="Connector1/AO7"}) -> ()  [unwired: 1 in]
            "Actual Analog Output Loop Period (usec)" <- w339
          }
        }
      }
      n107 = node-c288() -> (w100:T31)  [unwired: 1 in]
      n108 = timed-loop "EST APU Loop" {
        timing: w98 -> [_]
        timing-out: [_] -> w97
        tunnel: w96 -> [w101]
        stop <- _ stop-if-true
        n109 = call "Angle Processing Unit.vi"("settings.<user name>"="settings.apu 1", "register bus"=w101, "input.<user name>"="input.apu 1") -> ("output.<user name>"=→"output.apu 1":T26)  [unwired: 8 in]
      }
      n110 = timed-loop "Digital High Speed Loop" {
        timing: w100 -> [_]
        timing-out: [_] -> w99
        tunnel: w96 -> [w113]
        tunnel: w93 -> [w112]
        tunnel: w92 -> [w111]
        tunnel: w91 -> [w110]
        tunnel: w90 -> [w109]
        stop <- _ stop-if-true
        n111 = flat-sequence "Timing Control" {
          tunnel: w113 -> [w212]
          tunnel: w112 -> [w213]
          tunnel: w111 -> [w209]
          tunnel: w110 -> [w206]
          tunnel: w109 -> [w203]
          frame #0 {
            n112 = call "Directional Speed Sensor.vi"("load data"=w203, "settings.<user name>"="settings.Crank", "register bus"=w212, "input.<user name>"="input.Crank") -> ("digial output"=w195:bool)  [unwired: 7 in]
            n113 = call "Digital Pattern Generation.vi"("load data"=w213, "settings.<user name>"="settings.Intake CAM 1", "register bus"=w212, "input.<user name>"="input.Intake CAM 1") -> ("digial output"=w200:bool)  [unwired: 7 in]
            n114 = call "Digital Pattern Generation.vi"("load data"=w209, "settings.<user name>"="settings.Exhaust CAM 1", "register bus"=w212, "input.<user name>"="input.Exhaust CAM 1") -> ("digial output"=w199:bool)  [unwired: 7 in]
            n115 = call "Digital Pattern Generation.vi"("load data"=w206, "settings.<user name>"="settings.Crank_Temp", "register bus"=w212, "input.<user name>"="input.Crank_Temp") -> ("digial output"=w196:bool)  [unwired: 7 in]
            n116 = call "PWM.Generate.Digital.vi"("Settings"="PWM Out 1.Settings") -> ("Output"=w202:bool)  [unwired: 10 in]
            n117 = call "PWM.Generate.Digital.vi"("Settings"="PWM Out 2.Settings") -> ("Output"=w201:bool)  [unwired: 10 in]
            n118 = call "Digital_Input_8Channels.vi"("IO"=T34 {"DI 0"="Connector1/DIO0", "DI 1"="Connector1/DIO1", "DI 2"="Connector1/DIO6", "DI 3"="Connector1/DIO2", "DI 4"="Connector1/DIO4", "DI 5"="Connector1/DIO5", "DI 6"="Connector1/DIO3", "DI 7"="Connector1/DIO7"}) -> ("States"=w126:bool[])
            "Connector1 DIO Bank0.Monitor" <- w126
            n119 = call "WSS.Generate.Digital.vi"("Settings"="Front Driver WS.Settings") -> ("Bit1"=w190:bool, "Bit0"=w191:bool)  [unwired: 8 in, 1 out]
            n120 = call "WSS.Generate.Digital.vi"("Settings"="Front Passenger WS.Settings") -> ("Bit1"=w187:bool, "Bit0"=w188:bool)  [unwired: 8 in, 1 out]
            n121 = call "WSS.Generate.Digital.vi"("Settings"="Rear Driver WS.Settings") -> ("Bit1"=w184:bool, "Bit0"=w185:bool)  [unwired: 8 in, 1 out]
            n122 = call "WSS.Generate.Digital.vi"("Settings"="Read Passenger WS.Settings") -> ("Bit1"=w181:bool, "Bit0"=w182:bool)  [unwired: 8 in, 1 out]
            n123 = call "Digital_Input_8Channels.vi"("IO"=T34 {"DI 0"="Connector0/DIO16", "DI 1"="Connector0/DIO17", "DI 2"="Connector0/DIO18", "DI 3"="Connector0/DIO19", "DI 4"="Connector0/DIO20", "DI 5"="Connector0/DIO21", "DI 6"="Connector0/DIO22", "DI 7"="Connector0/DIO23"}) -> ("States"=w173:bool[])
            "Connector0 DIO Bank2.Monitor" <- w173
            n124 = Index Array(array=w126) -> (element #1=w124:bool, element #2=w123:bool, element #3=w122:bool, element #4=w119:bool, element #5=w118:bool, element #6=w117:bool, element #7=→"Check The Channel 1":bool, element #8=→"Check The Channel 2":bool)  [unwired: 8 in]
            n125 = call "QuadratureEncoder.Measure.Digital.vi"("Z"=w122, "B"=w123, "A"=w124, "Settings"="Measured Engine Position.Settings") -> ("Measurement"=→"Measured Engine Position.Measure":T1)  [unwired: 7 in]
            n126 = call "QuadratureEncoder.Measure.Digital.vi"("Z"=w117, "B"=w118, "A"=w119, "Settings"="Measured CAM Position.Settings") -> ("Measurement"=→"Measured CAM Position.Measure":T1)  [unwired: 7 in]
            n127 = Build Array(w202, w201, w200, w199, "Key", "Switch", w196, w195) -> (w193:bool[])
            "Connector0 DIO Bank0.Monitor" <- w193
            n128 = Build Array(w191, w190) -> (w180:bool[])
            n129 = Build Array(w188, w187) -> (w179:bool[])
            n130 = Build Array(w185, w184) -> (w178:bool[])
            n131 = Build Array(w182, w181) -> (w177:bool[])
            n132 = Index Array(array=w173) -> (element #1=→"Relay State":bool, element #2=→"Switch State":bool, element #3=→"Key State":bool, element #4=w168:bool, element #5=w165:bool, element #6=w162:bool, element #7=w150:bool, element #8=w138:bool)  [unwired: 8 in]
            n133 = call "Digital_Output_8Channels.vi"("States"=w193, "IO"=T36 {"DO 0"="Connector0/DIO0", "DO 1"="Connector0/DIO1", "DO 2"="Connector0/DIO2", "DO 3"="Connector0/DIO3", "DO 4"="Connector0/DIO4", "DO 5"="Connector0/DIO5", "DO 6"="Connector0/DIO6", "DO 7"="Connector0/DIO7"}) -> ()  [unwired: 1 in]
            n134 = Build Array (concatenate)(w180, w179, w178, w177) -> (w175:bool[])
            "Connector0 DIO Bank1.Monitor" <- w175
            n135 = call "Digital_Output_8Channels.vi"("States"=w175, "IO"=T36 {"DO 0"="Connector0/DIO8", "DO 1"="Connector0/DIO9", "DO 2"="Connector0/DIO10", "DO 3"="Connector0/DIO11", "DO 4"="Connector0/DIO12", "DO 5"="Connector0/DIO13", "DO 6"="Connector0/DIO14", "DO 7"="Connector0/DIO15"}) -> ()  [unwired: 1 in]
            n136 = call "PWM.Measure.Digital.vi"("State"=w165, "Settings"="PWM IN 2.Settings") -> ("Measurement"=→"PWM IN 2.Measure":T6)  [unwired: 8 in, 1 out]
            n137 = call "PWM.Measure.Digital.vi"("State"=w168, "Settings"="PWM IN 1.Settings") -> ("Measurement"=→"PWM IN 1.Measure":T6)  [unwired: 8 in, 1 out]
            n138 = call-poly "Measure Events.vi"("settings.<user name>"="settings.Cyl Inj 1", "register bus"=w212, "event"=w162) -> ("measured data"=w159:T43, "status.<user name>"=→"status.Cyl Inj 1":T4)  [unwired: 7 in]
            n139 = call-poly "Measure Events.vi"("settings.<user name>"="settings.Cyl Inj 2", "register bus"=w212, "event"=w150) -> ("measured data"=w147:T43, "status.<user name>"=→"status.Cyl Inj 2":T4)  [unwired: 7 in]
            n140 = call-poly "Measure Events.vi"("settings.<user name>"="settings.Cyl Inj 3", "register bus"=w212, "event"=w138) -> ("measured data"=w135:T43, "status.<user name>"=→"status.Cyl Inj 3":T4)  [unwired: 7 in]
            n141 = call "Capture Event.vi"("event # to capture"=T35 1, "measured data"=w159) -> ("capture.<user name>"=→"capture.Cyl Inj 1.Event 1":T3)  [unwired: 9 in]
            n142 = call "Capture Event.vi"("event # to capture"=T35 2, "measured data"=w159) -> ("capture.<user name>"=→"capture.Cyl Inj 1.Event 2":T3)  [unwired: 9 in]
            n143 = call "Capture Event.vi"("event # to capture"=T35 3, "measured data"=w159) -> ("capture.<user name>"=→"capture.Cyl Inj 1.Event 3":T3)  [unwired: 9 in]
            n144 = call "Capture Event.vi"("event # to capture"=T35 4, "measured data"=w159) -> ("capture.<user name>"=→"capture.Cyl Inj 1.Event 4":T3)  [unwired: 9 in]
            n145 = call "Capture Event.vi"("event # to capture"=T35 1, "measured data"=w147) -> ("capture.<user name>"=→"capture.Cyl Inj 2.Event 1":T3)  [unwired: 9 in]
            n146 = call "Capture Event.vi"("event # to capture"=T35 2, "measured data"=w147) -> ("capture.<user name>"=→"capture.Cyl Inj 2.Event 2":T3)  [unwired: 9 in]
            n147 = call "Capture Event.vi"("event # to capture"=T35 3, "measured data"=w147) -> ("capture.<user name>"=→"capture.Cyl Inj 2.Event 3":T3)  [unwired: 9 in]
            n148 = call "Capture Event.vi"("event # to capture"=T35 4, "measured data"=w147) -> ("capture.<user name>"=→"capture.Cyl Inj 2.Event 4":T3)  [unwired: 9 in]
            n149 = call "Capture Event.vi"("event # to capture"=T35 4, "measured data"=w135) -> ("capture.<user name>"=→"capture.Cyl Inj 3.Event 4":T3)  [unwired: 9 in]
            n150 = call "Capture Event.vi"("event # to capture"=T35 1, "measured data"=w135) -> ("capture.<user name>"=→"capture.Cyl Inj 3.Event 1":T3)  [unwired: 9 in]
            n151 = call "Capture Event.vi"("event # to capture"=T35 2, "measured data"=w135) -> ("capture.<user name>"=→"capture.Cyl Inj 3.Event 2":T3)  [unwired: 9 in]
            n152 = call "Capture Event.vi"("event # to capture"=T35 3, "measured data"=w135) -> ("capture.<user name>"=→"capture.Cyl Inj 3.Event 3":T3)  [unwired: 9 in]
          }
        }
      }
      n153 = node-c288 ("Output Node")(w97) -> ()
      n154 = node-c288 ("Output Node")(w99) -> ()
    }
  }
